vi "Read Data.vi"(8 "error in (no error)":errorcluster, 10 "LogicName":string, 11 "PLC_Module in":refnum<class "PLC_Module.lvclass">) -> (0 "error out":errorcluster, 2 "Data":variant, 3 "PLC_Module out":refnum<class "PLC_Module.lvclass">)   [LabVIEW 2025, in "PLC_Module.lvlib" / "PLC_Module.lvclass"]
uses:
  PLC_Module.lvclass
  PLC_Module.lvclass/PLC_Module.ctl
  PLC_Abstr/PLC_Abstr Messages/Read Data Msg/Read Data Msg.lvclass/Read Data Msg.ctl
  <vilib>/ActorFramework/Message Enqueuer/Message Enqueuer.lvclass/Message Enqueuer.ctl
  Read Configuration.vi
  <vilib>/ActorFramework/Message Enqueuer/Enqueue.vi
  PLC_Abstr/PLC_Abstr Messages/Read Data Msg/Read Data Msg.lvclass
  C:/Program Files (x86)/National Instruments/LabVIEW 2025/vi.lib/ActorFramework/Message/Message.lvclass
  <vilib>/ActorFramework/Message Priority Queue/Priority Enqueue.vi
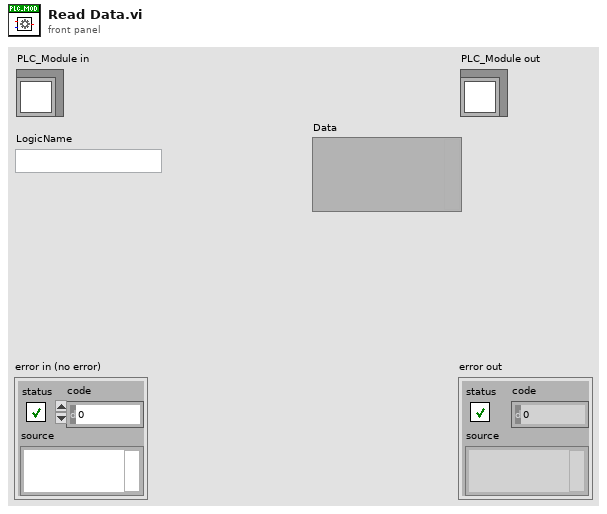
[diagram p1: front panel]
types:
  T1 = typedef "PLC_Module.lvlib/PLC_Module.lvclass/PLC_Data_Config.ctl" = map{string, cluster{"Config":T2, "Value":string}}
  T2 = typedef "PLC_Module.lvlib/PLC_Module.lvclass/PLC_Data.ctl" = cluster{"StartAddress":u32, "Direction":enum16{"PC->PLC", "PLC->PC"}, "DataType":T3, "DefaultValue":string, "Description":string}
  T3 = typedef "PLC_Module.lvlib/PLC_Module.lvclass/PLC_Data_Type.ctl" = enum16{"U8", "U32", "U32_Array", "String"}
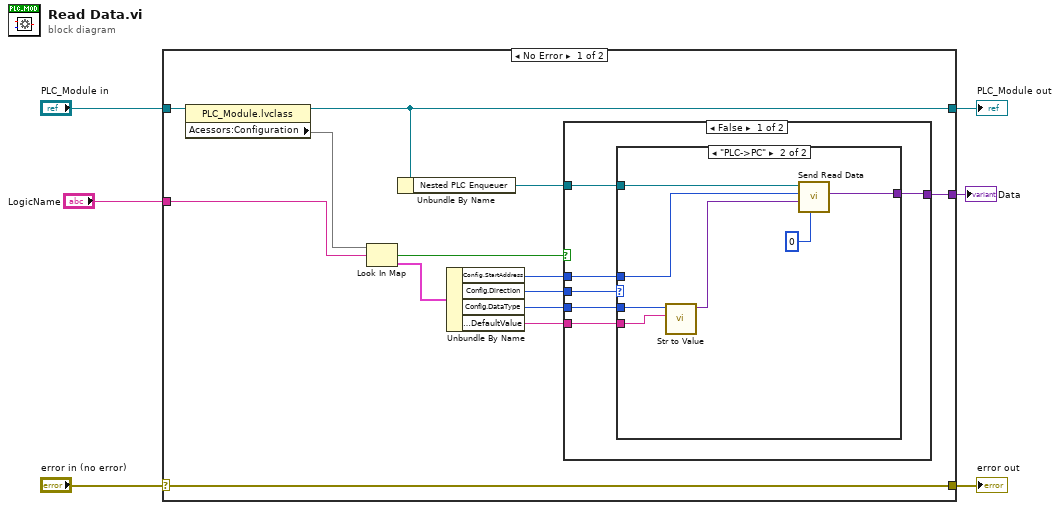
[diagram p0: block diagram]
diagram:
  n1 = case shown="No Error" "error in (no error)" {
    selector: "error in (no error)" -> [w19 w34]
    tunnel: [w19 w34] -> w5
    tunnel: [w15 w33] -> w3
    tunnel: "PLC_Module in" -> [w18 w33]
    tunnel: "LogicName" -> [w16 _]
    tunnel: [w7 _] -> w1
    frame No Error {
      n2 = property class="PLC_Module.lvclass"(reference=w18) -> (reference out=w15:refnum<class "PLC_Module.lvclass">, "Acessors:Configuration"=w17:T1)  [unwired: 1 in, 1 out]
      n3 = Look In Map(map=w17, key=w16) -> (key not found?=w13:bool, value=w12:cluster{"Config":T2, "Value":string})  [unwired: 1 in]
      n4 = Unbundle By Name(w15) -> ("Nested PLC Enqueuer"=w14:refnum<class "Message Enqueuer.lvclass">)
      n5 = Unbundle By Name(w12) -> ("Config.StartAddress"=w11:u32, "Config.Direction"=w10:enum16{"PC->PLC", "PLC->PC"}, "Config.DataType"=w9:T3, "Config.DefaultValue"=w8:string)
      n6 = case shown="False" w13 {
        tunnel: w14 -> [w25 _]
        tunnel: w11 -> [w24 _]
        tunnel: w10 -> [w23 _]
        tunnel: w9 -> [w22 _]
        tunnel: w8 -> [w21 _]
        tunnel: [w20 _] -> w7
        frame False {
          n7 = case shown="\"PLC->PC\"" w23 {
            tunnel: w25 -> [_ w32]
            tunnel: w24 -> [_ w31]
            tunnel: w22 -> [_ w28]
            tunnel: w21 -> [_ w27]
            tunnel: [_ w29] -> w20
            frame "PC->PLC", Default {
            }
            frame "PLC->PC" {
              n8 = call "Str to Value.vi"("DefaultValue"=w27, "DataType"=w28) -> ("Variant"=w26:variant)  [unwired: 8 in, 1 out]
              n9 = call "Send Read Data.vi"("Data Block"=u16 0, "Default Data"=w26, "Start Address"=w31, "Message Enqueuer"=w32) -> ("Data"=w29:variant)  [unwired: 5 in, 2 out]
            }
          }
        }
        frame True {
        }
      }
    }
    frame Error {
    }
  }
  "error out" <- w5
  "PLC_Module out" <- w3
  "Data" <- w1
